vi "PH_OceanOpticsSpectrometer.Read Spectra.vi"(0 "i ref in":refnum<vi>, 5 "error in (no error)":errorcluster) -> (14 "i ref out":refnum<vi>, 19 "error out":errorcluster)   [LabVIEW 2014, in "PH_OceanOpticsSpectrometer.lvlib"]
doc: "This VI reads the spectra out of the device and indicates the data."
uses:
  PH_OceanOpticsSpectrometer.lvlib
  PH_Basics/PH_Common/PH_Common.lvlib
  instr.lib/OceanOpticsSpectrometer/Ocean Optics 2000 4000 - Driver np.lvlib
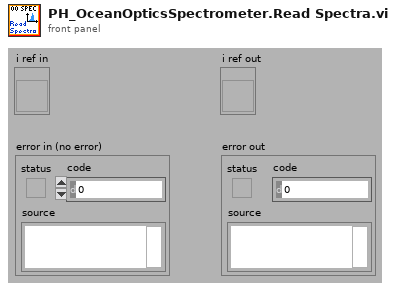
[diagram p1: front panel]
types:
  T1 = typedef "PH_OceanOpticsSpectrometer.lvlib/PH_OceanOpticsSpectrometer.i attribute.ctl" = cluster{"GUI Refs":cluster{"Delete":refnum<vi>, "Spectrum":refnum<vi>, "Display Width":refnum<vi>, "Display Center":refnum<vi>, "Save":refnum<vi>, "Integration time":refnum<vi>, "center wavelength":refnum<vi>, "width":refnum<vi>, "Wanted Trigger Mode":refnum<vi>, "Current Trigger Mode":refnum<vi>, "Trigger Info":refnum<vi>, "Model":refnum<vi>, "Driver":refnum<vi>, "Firmware":refnum<vi>}, "Display":cluster{"Width":dbl, "Center":dbl}, "VISA resource name":refnum<visa-resource-name>, "Integration time [ms]":cluster{"Current Value":u16, "Wanted Value":u16}, "Trigger":cluster{"Current value":T2, "Wanted value":T2}, "Default VISA Timeout":u32, "Last Data":cluster{"Wavelength Bins":dbl[], "Spectrum by Pixels":dbl[]}}
  T2 = typedef "PH_OceanOpticsSpectrometer.lvlib/PH_OceanOpticsSpectrometer.Trigger.ctl" = enum32{"External", "Normal"}
  T3 = cluster{"Wavelength Bins":dbl[], "Spectrum by Pixels":dbl[]}
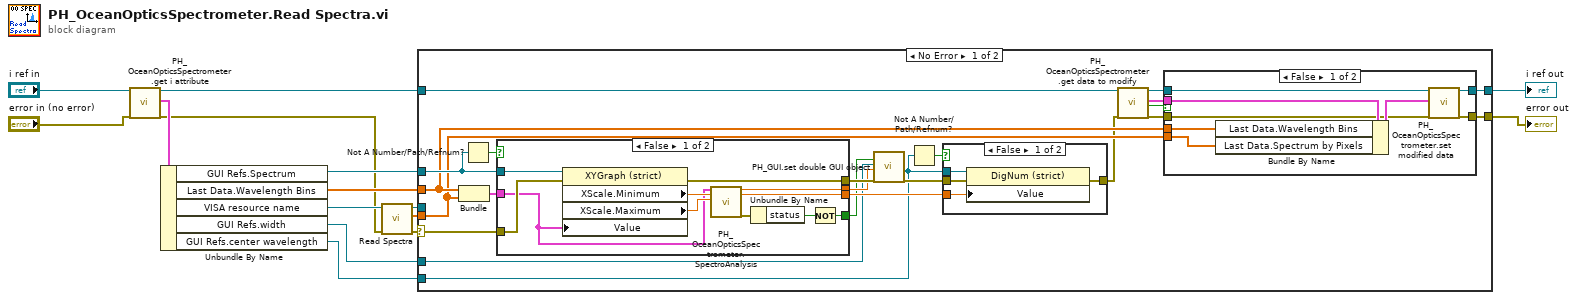
[diagram p0: block diagram]
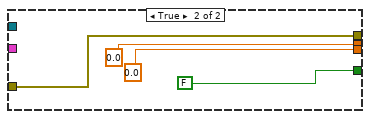
[diagram p4: hidden frame]
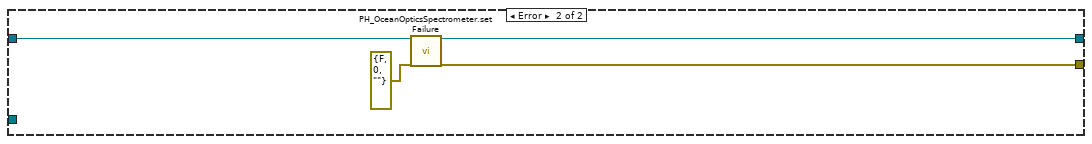
[diagram p5: hidden frame]
diagram:
  n1 = call "PH_OceanOpticsSpectrometer.get i attribute.vi"("i ref in"="i ref in", "error in (no error)"="error in (no error)") -> ("i ref out"=w5:refnum<vi>, "i attribute"=w12:T1, "error out"=w4:errorcluster)  [unwired: 15 in]
  n2 = Unbundle By Name(w12) -> ("GUI Refs.Spectrum"=w7:refnum<vi>, "Last Data.Wavelength Bins"=w13:dbl[], "VISA resource name"=w6:refnum<visa-resource-name>, "GUI Refs.width"=w14:refnum<vi>, "GUI Refs.center wavelength"=w15:refnum<vi>)
  n3 = call "Read Spectra.vi"("error in (no error)"=w4, "VISA resource name"=w6) -> ("error out"=w3:errorcluster, "Spectrum by Pixels"=w2:dbl[], "VISA resource name out"=w1:refnum<visa-resource-name>)  [unwired: 7 in]
  n4 = case shown="No Error" w3 {
    selector: w3 -> [w37 _]
    tunnel: w2 -> [w19 _]
    tunnel: w13 -> [w20 _]
    tunnel: w7 -> [w36 _]
    tunnel: [w23 w69] -> w11
    tunnel: w14 -> [w18 _]
    tunnel: w15 -> [w17 _]
    tunnel: w5 -> [w22 w71]
    tunnel: [w21 w70] -> w9
    tunnel: w1 -> [_ _]
    frame No Error {
      n5 = Bundle("Wavelength Bins"=w20, "Spectrum by Pixels"=w19) -> (w34:T3)  [unwired: 1 in]
      n6 = Not A Number/Path/Refnum?(number/path/refnum=w36) -> (NaN/Path/Refnum?=w35:bool)
      n7 = case shown="False" w35 {
        tunnel: w37 -> [w63 w67]
        tunnel: w36 -> [w62 _]
        tunnel: [w54 w67] -> w33
        tunnel: w34 -> [w53 _]
        tunnel: [w59 0.0 ("width")] -> w32
        tunnel: [w58 sgl 0.0 ("center wavelength")] -> w30
        tunnel: [w55 FALSE] -> w28
        frame False {
          n8 = property class="XYGraph (strict)"(reference=w62, error in=w63, "Value"=w53) -> (error out=w54:errorcluster, "XScale.Minimum"=w61:dbl, "XScale.Maximum"=w60:dbl)  [unwired: 1 out]
          n9 = call "PH_OceanOpticsSpectrometer.SpectroAnalysis.vi"("Spectrum"=w53, "lower Limit"=w61, "upper Limit"=w60) -> ("width"=w59:dbl, "center wavelength"=w58:sgl, "error out"=w57:errorcluster)  [unwired: 14 in]
          n10 = Unbundle By Name(w57) -> ("status"=w56:bool)
          n11 = Not(x=w56) -> (.not. x?=w55:bool)
        }
        frame True {
        }
      }
      n12 = call "PH_GUI.set double GUI object.vi"("visible (true)"=w28, "GUI object Ref"=w18, "value"=w32, "error in (no error)"=w33) -> ("error out"=w29:errorcluster)  [unwired: 15 in]
      n13 = Not A Number/Path/Refnum?(number/path/refnum=w17) -> (NaN/Path/Refnum?=w31:bool)
      n14 = case shown="False" w31 {
        tunnel: w17 -> [w50 _]
        tunnel: w29 -> [w51 w52]
        tunnel: [w49 w52] -> w16
        tunnel: w30 -> [w48 _]
        frame False {
          n15 = property class="DigNum (strict)"(reference=w50, error in=w51, "Value"=w48) -> (error out=w49:errorcluster)  [unwired: 1 out]
        }
        frame True {
        }
      }
      n16 = call "PH_OceanOpticsSpectrometer.get data to modify.vi"("i ref in"=w22, "error in (no error)"=w16) -> ("i ref out"=w25:refnum<vi>, "i attribute"=w27:T1, "timed out"=w26:bool, "error out"=w24:errorcluster)  [unwired: 14 in]
      n17 = case shown="False" w26 {
        tunnel: w24 -> [w40 w46]
        tunnel: [w41 w46] -> w23
        tunnel: w25 -> [w45 w47]
        tunnel: [w44 w47] -> w21
        tunnel: w27 -> [w42 _]
        tunnel: w20 -> [w39 _]
        tunnel: w19 -> [w38 _]
        frame False {
          n18 = Bundle By Name(cluster=w42, "Last Data.Wavelength Bins"=w39, "Last Data.Spectrum by Pixels"=w38) -> (w43:T1)
          n19 = call "PH_OceanOpticsSpectrometer.set modified data.vi"("i ref in"=w45, "i attribute"=w43, "error in (no error)"=w40) -> ("i ref out"=w44:refnum<vi>, "error out"=w41:errorcluster)  [unwired: 15 in]
        }
        frame True {
        }
      }
    }
    frame Error {
      n20 = call "PH_OceanOpticsSpectrometer.set Failure.vi"("i ref in"=w71, "error IO"=errorcluster {"status"=FALSE, "code"=0, "source"=""}) -> ("i ref out"=w70:refnum<vi>, "error out"=w69:errorcluster)  [unwired: 16 in]
    }
  }
  "error out" <- w11
  "i ref out" <- w9
